vi "tm3samp_06_framerate_wVision.vi"() -> ()   [LabVIEW 2011]
panel:
  out "Display":T1(plugin-control)
  out "Software FPS":dbl
  out "Camera FPS":dbl
  out "Camera Serial":string
  out "Camera Version":string
  out "Camera Model":string
  out "SMD":dbl
  in  "Scan Mode":dbl min=1.0 max=2.0 step=1.0
  in  "Exposure":dbl min=0.0010036691729323308 max=10.000004210526315 step=1e-08
  out "EXP":dbl
  out "SVW":i32
  out "SHW":i32
  out "SVO":i32
  out "SHO":i32
  in  "V Width":i32 min=4 max=1028 step=4
  in  "V Offset":i32 min=0 max=2044 step=4
  in  "H Width":i32 min=4 max=2048 step=4
  in  "H Offset":i32 min=0 max=0 step=4
  in  "Binning":u16(ring)=1 items=["1x1"=1, "2x2"=2, "4x4"=4]
  out "Elapsed Time":u32
  out "Total Frames":i32
  in  "Display":bool=TRUE
  out "error out":errorcluster
  in  "stop":bool
  # "This example displays the frame rate\nof the camera.  Changing the resolution\nof the camera or displaying the images\nwill affect the frame rate."
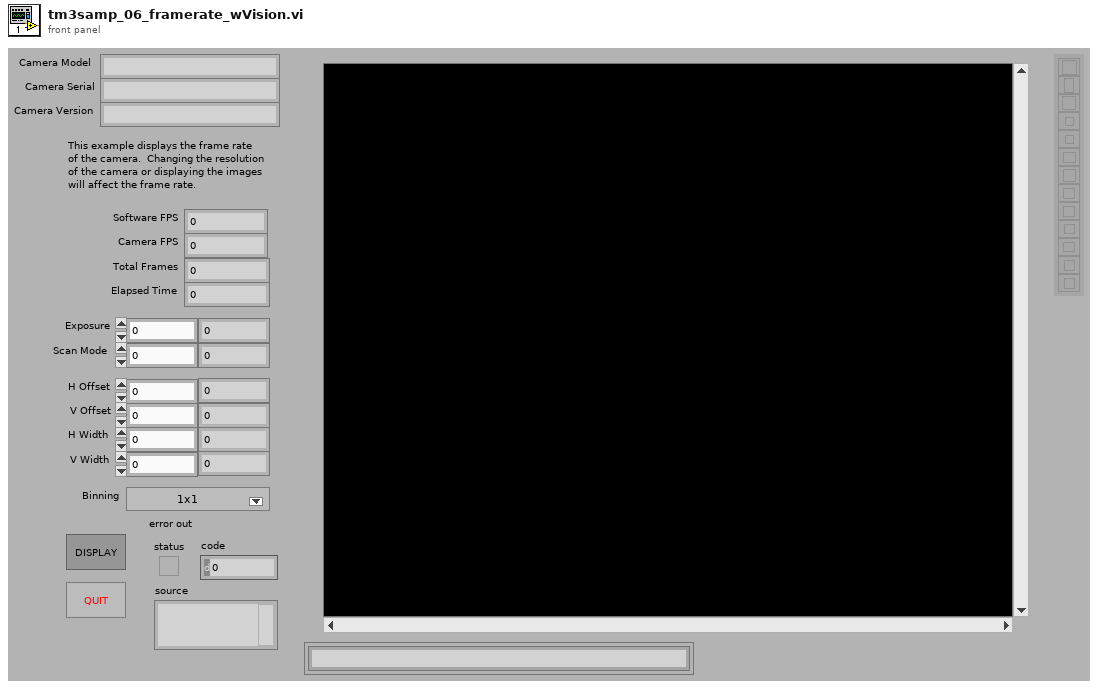
[diagram p1: front panel]
types:
  T1 = typedef "IMAQ Image.ctl" = refnum<image>
  T2 = typedef "Image Type" = u32
  T3 = cluster{"Model":string, "Camera ID":string, "Firmware":string}
  T4 = cluster{"Value":i32, "Minimum":i32, "Maximum":i32, "Increment":i32}
  T5 = cluster{"height":u32, "width":u32, "datatype":u32}
  T6 = cluster{"H Offset":i32, "V Offset":i32, "H Width":i32, "V Width":i32}
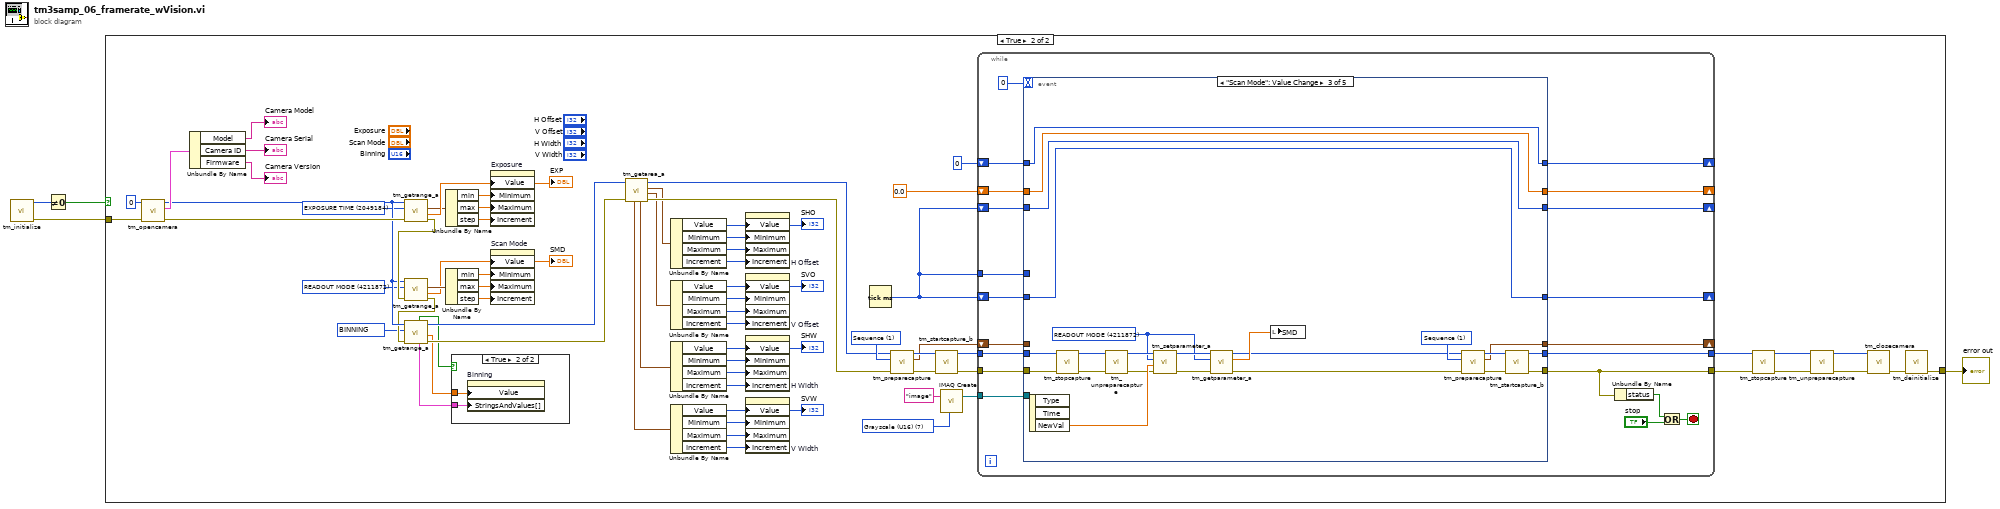
[diagram p0: block diagram]
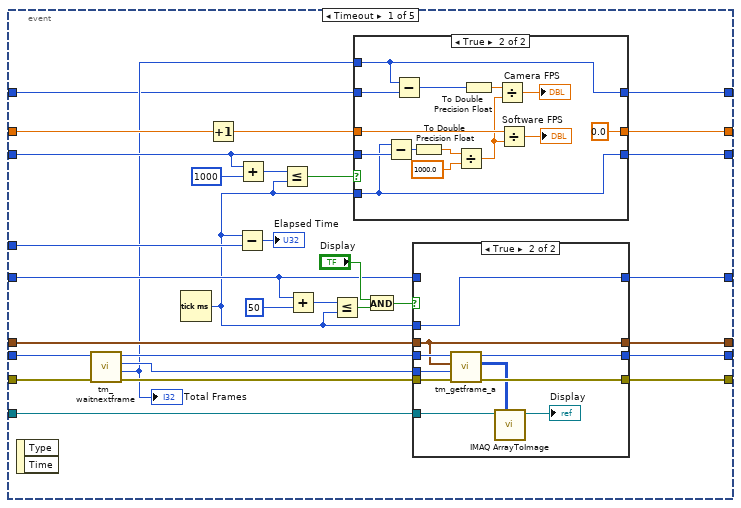
[diagram p4: hidden frame]
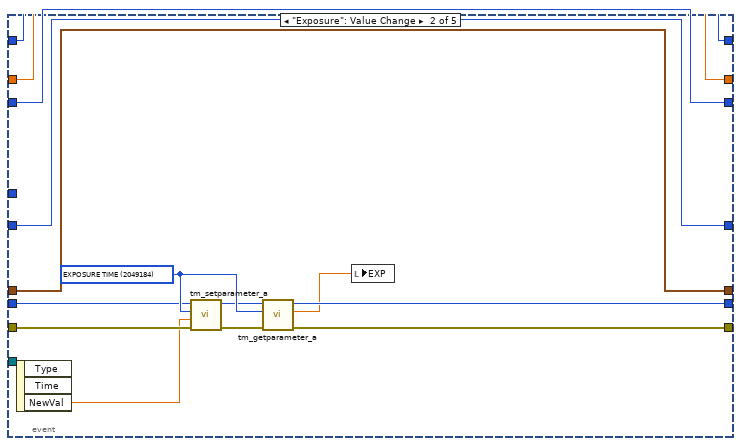
[diagram p7: hidden frame]
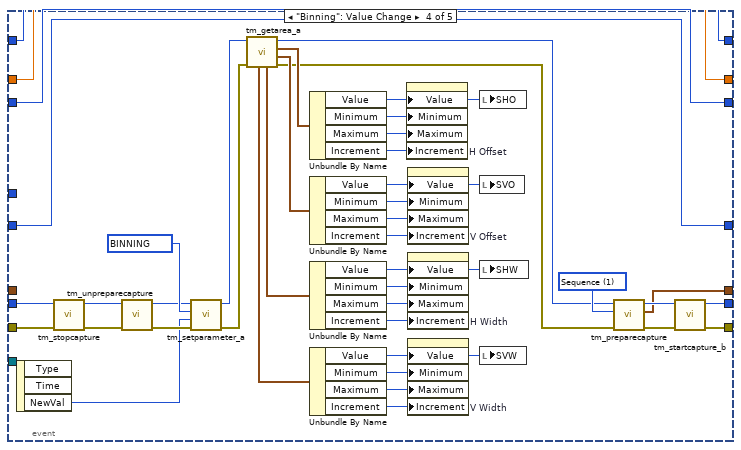
[diagram p8: hidden frame]
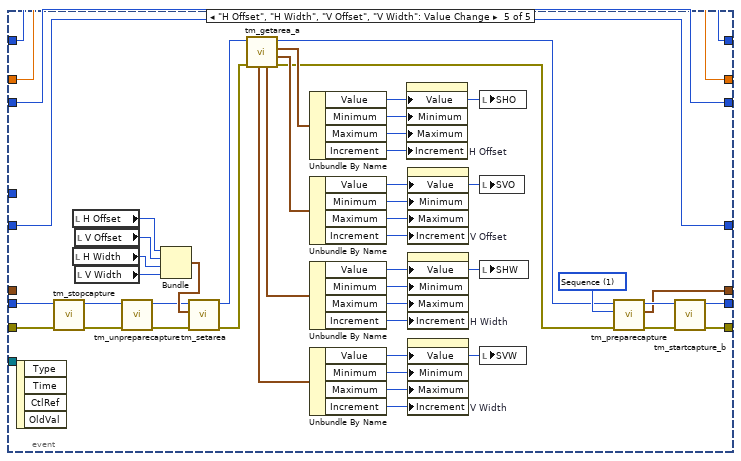
[diagram p9: hidden frame]
diagram:
  n1 = call <userlib>:"tm_initialize.vi"() -> ("error out"=w2:errorcluster, "Number Of Cameras"=w1:u32)  [unwired: 8 in, 2 out]
  n2 = Not Equal To 0?(x=w1) -> (x != 0?=w4:bool)
  n3 = case shown="True" w4 {
    tunnel: [w5 w72] -> w3
    tunnel: w2 -> [w5 w75]
    frame False {
    }
    frame True {
      w7 = T2 7 items=["Grayscale (U8)", "Grayscale (I16)", "Grayscale (SGL)", "Complex (CSG)", "RGB (U32)", "HSL (U32)", "RGB (U64)", "Grayscale (U16)"] ("Image Type")
      w9 = u32 2049184 items=["BINNING"=4215968, "BITS PER CHANNEL"=4342976, "ACTIVE VIEW INDEX"=4343136, "CCD MODE"=4212384, "SENSOR MODE"=4212128, "READOUT MODE"=4211872, "EXPOSURE TIME"=2049184, "CONTRAST GAIN"=3163312, "CONTRAST OFFSET"=3163328, "LIGHT MODE"=2114720, "SENSITIVITY"=2114992, "WHITE BALANCE"=3163568, "PHOTON IMAGING MODE"=2115200, "HIGH DYNAMIC RANGE MODE"=3163360, "TRIGGER SOURCE"=1066144, "TRIGGER ACTIVE"=1066160, "TRIGGER MODE"=1066400, "TRIGGER POLARITY"=1066416, "TRIGGER GLOBAL EXPOSURE"=2049680, "FIRST TRIGGER BEHAVIOR"=2049696, "TRIGGER TIMES"=1066448, "OUTPUT TRIGGER POLARITY"=1852592, "OUTPUT TRIGGER DELAY"=1852624, "OUTPUT TRIGGER PERIOD"=1852640, "TEMPERATURE"=2115232, "TEMPERATURE TARGET"=2115264, "SENSOR COOLER FAN"=2115296, "MECHANICAL SHUTTER"=2115488, "BACK FOCUS POSITION"=8422304, "FRAMEBUNDLE MODE"=4346784, "FRAMEBUNDLE NUMBER"=4346800, "LINEBUNDLE HEIGHT"=4212192, "TRIGGER CONNECTOR"=1066432, "IMAGE PIXEL TYPE"=4343296, "OUTPUT TRIGGER KIND"=1852656, "READOUT DIRECTION"=4211904, "CHANNEL SYNC"=1852352] ("Parameter")
      w10 = u32 4211872 items=["BINNING"=4215968, "BITS PER CHANNEL"=4342976, "ACTIVE VIEW INDEX"=4343136, "CCD MODE"=4212384, "SENSOR MODE"=4212128, "READOUT MODE"=4211872, "EXPOSURE TIME"=2049184, "CONTRAST GAIN"=3163312, "CONTRAST OFFSET"=3163328, "LIGHT MODE"=2114720, "SENSITIVITY"=2114992, "WHITE BALANCE"=3163568, "PHOTON IMAGING MODE"=2115200, "HIGH DYNAMIC RANGE MODE"=3163360, "TRIGGER SOURCE"=1066144, "TRIGGER ACTIVE"=1066160, "TRIGGER MODE"=1066400, "TRIGGER POLARITY"=1066416, "TRIGGER GLOBAL EXPOSURE"=2049680, "FIRST TRIGGER BEHAVIOR"=2049696, "TRIGGER TIMES"=1066448, "OUTPUT TRIGGER POLARITY"=1852592, "OUTPUT TRIGGER DELAY"=1852624, "OUTPUT TRIGGER PERIOD"=1852640, "TEMPERATURE"=2115232, "TEMPERATURE TARGET"=2115264, "SENSOR COOLER FAN"=2115296, "MECHANICAL SHUTTER"=2115488, "BACK FOCUS POSITION"=8422304, "FRAMEBUNDLE MODE"=4346784, "FRAMEBUNDLE NUMBER"=4346800, "LINEBUNDLE HEIGHT"=4212192, "TRIGGER CONNECTOR"=1066432, "IMAGE PIXEL TYPE"=4343296, "OUTPUT TRIGGER KIND"=1852656, "READOUT DIRECTION"=4211904, "CHANNEL SYNC"=1852352] ("Parameter")
      w11 = u32 4215968 items=["BINNING"=4215968, "BITS PER CHANNEL"=4342976, "ACTIVE VIEW INDEX"=4343136, "CCD MODE"=4212384, "SENSOR MODE"=4212128, "READOUT MODE"=4211872, "EXPOSURE TIME"=2049184, "CONTRAST GAIN"=3163312, "CONTRAST OFFSET"=3163328, "LIGHT MODE"=2114720, "SENSITIVITY"=2114992, "WHITE BALANCE"=3163568, "PHOTON IMAGING MODE"=2115200, "HIGH DYNAMIC RANGE MODE"=3163360, "TRIGGER SOURCE"=1066144, "TRIGGER ACTIVE"=1066160, "TRIGGER MODE"=1066400, "TRIGGER POLARITY"=1066416, "TRIGGER GLOBAL EXPOSURE"=2049680, "FIRST TRIGGER BEHAVIOR"=2049696, "TRIGGER TIMES"=1066448, "OUTPUT TRIGGER POLARITY"=1852592, "OUTPUT TRIGGER DELAY"=1852624, "OUTPUT TRIGGER PERIOD"=1852640, "TEMPERATURE"=2115232, "TEMPERATURE TARGET"=2115264, "SENSOR COOLER FAN"=2115296, "MECHANICAL SHUTTER"=2115488, "BACK FOCUS POSITION"=8422304, "FRAMEBUNDLE MODE"=4346784, "FRAMEBUNDLE NUMBER"=4346800, "LINEBUNDLE HEIGHT"=4212192, "TRIGGER CONNECTOR"=1066432, "IMAGE PIXEL TYPE"=4343296, "OUTPUT TRIGGER KIND"=1852656, "READOUT DIRECTION"=4211904, "CHANNEL SYNC"=1852352] ("Parameter")
      w70 = 1 items=["Snap", "Sequence"] ("Capture mode")
      n4 = call <userlib>:"tm_opencamera.vi"("error in (no error)"=w75, "Camera Index"=u32 0) -> ("error out"=w24:errorcluster, "Camera Details"=w28:T3, "Handle out"=w18:u32)  [unwired: 7 in]
      n5 = Unbundle By Name(w28) -> ("Model"=→"Camera Model":string, "Camera ID"=→"Camera Serial":string, "Firmware"=→"Camera Version":string)
      n6 = call <userlib>:"tm_getrange_a.vi"("error in (no error)"=w24, "Parameter"=w9, "Handle in"=w18) -> ("error out"=w21:errorcluster, "default"=w23:dbl, "Range"=w22:cluster{"min":dbl, "max":dbl, "step":dbl})  [unwired: 2 in, 4 out]
      "EXP" <- w23
      n7 = call <userlib>:"tm_getrange_a.vi"("error in (no error)"=w21, "Parameter"=w10, "Handle in"=w18) -> ("error out"=w17:errorcluster, "default"=w19:dbl, "Range"=w20:cluster{"min":dbl, "max":dbl, "step":dbl})  [unwired: 2 in, 4 out]
      "SMD" <- w19
      n8 = call <userlib>:"tm_getrange_a.vi"("error in (no error)"=w17, "Parameter"=w11, "Handle in"=w18) -> ("error out"=w16:errorcluster, "default"=w13:dbl, "Handle out"=w15:u32, "Value Names"=w12:cluster{"Name":string, "Value":dbl}[], "Writable"=w14:bool)  [unwired: 2 in, 2 out]
      n9 = Unbundle By Name(w22) -> ("min"=w63:dbl, "max"=w62:dbl, "step"=w61:dbl)
      n10 = Unbundle By Name(w20) -> ("min"=w60:dbl, "max"=w59:dbl, "step"=w58:dbl)
      n11 = case shown="True" w14 {
        tunnel: w12 -> [_ w77]
        tunnel: w13 -> [_ w76]
        frame False {
        }
        frame True {
          n12 = property on="Binning" class="Ring (strict)"("Value"=w76, "StringsAndValues[]"=w77) -> ()  [unwired: 2 in, 2 out]
        }
      }
      n13 = property on="Exposure" class="DigNum (strict)"("Value"=w23, "Minimum"=w63, "Maximum"=w62, "Increment"=w61) -> ()  [unwired: 2 in, 2 out]
      n14 = property on="Scan Mode" class="DigNum (strict)"("Value"=w19, "Minimum"=w60, "Maximum"=w59, "Increment"=w58) -> ()  [unwired: 2 in, 2 out]
      n15 = call <userlib>:"tm_getarea_a.vi"("error in (no error)"=w16, "Handle in"=w15) -> ("error out"=w56:errorcluster, "V Offset"=w55:T4, "H Offset"=w34:T4, "Handle out"=w57:u32, "H Width"=w54:T4, "V Width"=w53:T4)  [unwired: 4 in]
      n16 = Unbundle By Name(w34) -> ("Value"=w33:i32, "Minimum"=w32:i32, "Maximum"=w31:i32, "Increment"=w30:i32)
      "SHO" <- w33
      n17 = Unbundle By Name(w55) -> ("Value"=w43:i32, "Minimum"=w52:i32, "Maximum"=w51:i32, "Increment"=w50:i32)
      "SVO" <- w43
      n18 = Unbundle By Name(w54) -> ("Value"=w42:i32, "Minimum"=w49:i32, "Maximum"=w48:i32, "Increment"=w47:i32)
      "SHW" <- w42
      n19 = Unbundle By Name(w53) -> ("Value"=w41:i32, "Minimum"=w46:i32, "Maximum"=w45:i32, "Increment"=w44:i32)
      "SVW" <- w41
      n20 = property on="H Offset" class="DigNum (strict)"("Value"=w33, "Minimum"=w32, "Maximum"=w31, "Increment"=w30) -> ()  [unwired: 2 in, 2 out]
      n21 = property on="V Offset" class="DigNum (strict)"("Value"=w43, "Minimum"=w52, "Maximum"=w51, "Increment"=w50) -> ()  [unwired: 2 in, 2 out]
      n22 = property on="H Width" class="DigNum (strict)"("Value"=w42, "Minimum"=w49, "Maximum"=w48, "Increment"=w47) -> ()  [unwired: 2 in, 2 out]
      n23 = property on="V Width" class="DigNum (strict)"("Value"=w41, "Minimum"=w46, "Maximum"=w45, "Increment"=w44) -> ()  [unwired: 2 in, 2 out]
      n24 = Tick Count (ms)() -> (millisecond timer value=w64:u32)
      n25 = call <userlib>:"tm_preparecapture.vi"("error in (no error)"=w56, "Capture mode"=w70, "Handle in"=w57) -> ("error out"=w68:errorcluster, "Buffer Info"=w65:T5, "Handle out"=w69:u32)  [unwired: 5 in, 1 out]
      n26 = call <userlib>:"tm_startcapture_b.vi"("error in (no error)"=w68, "Handle in"=w69) -> ("error out"=w67:errorcluster, "Handle out"=w66:u32)  [unwired: 8 in]
      n27 = call "IMAQ Create"("Image Name"="image", "Image Type"=w7) -> ("New Image"=w6:T1)  [unwired: 3 in, 1 out]
      n28 = while {
        tunnel: w67 -> [w86]
        tunnel: [w84] -> w40
        tunnel: [w83] -> w39
        shift-right: [w93] -> _
        shift-left: w64 -> [w91]
        shift-right: [w94] -> _
        shift-left: 0.0 -> [w92]
        shift-right: [w85] -> _
        shift-left: w64 -> [w89]
        tunnel: w66 -> [w87]
        tunnel: w64 -> [w90]
        shift-right: [w82] -> _
        shift-left: w65 -> [w88]
        shift-right: [w79] -> _
        shift-left: 0 -> [w80]
        tunnel: w6 -> [w78]
        stop <- w95 stop-if-true
        n29 = event shown="[2] \"Scan Mode\": Value Change" {
          selector: _ -> [_ _ _ _ _]
          dyn-events: _ -> [_ _ _ _ _]
          timeout: 0 -> [_ _ _ _ _]
          tunnel: [w103 w171 w194 w230 w275] -> w94
          tunnel: [w102 w172 w195 w231 w276] -> w93
          tunnel: w92 -> [w114 w171 w194 w230 w275]
          tunnel: w91 -> [w105 w172 w195 w231 w276]
          tunnel: w90 -> [w110 _ _ _ _]
          tunnel: w89 -> [w115 w173 w196 w238 w283]
          tunnel: w88 -> [w109 w170 _ _ _]
          tunnel: w87 -> [w117 w165 w191 w207 w245]
          tunnel: w86 -> [w116 w167 w190 w206 w244]
          tunnel: [w113 w173 w196 w238 w283] -> w85
          tunnel: [w112 w162 w185 w233 w278] -> w84
          tunnel: [w111 w160 w186 w234 w279] -> w83
          tunnel: [w108 w170 w184 w232 w277] -> w82
          tunnel: w80 -> [w100 w169 w183 w203 w239]
          tunnel: [w99 w169 w183 w203 w239] -> w79
          tunnel: w78 -> [w98 _ _ _ _]
          event Timeout {
            n30 = event-data() -> ()  [unwired: 1 in, 2 out]
            n31 = call <userlib>:"tm_waitnextframe.vi"("error in (no error)"=w116, "Handle in"=w117) -> ("error out"=w121:errorcluster, "Frame Count"=w101:i32, "Frame Index"=w120:i32, "Handle out"=w122:u32)  [unwired: 6 in]
            "Total Frames" <- w101
            n32 = Tick Count (ms)() -> (millisecond timer value=w107:u32)
            n33 = Increment(x=w114) -> (x+1=w104:dbl)
            n34 = Subtract(x=w107, y=w110) -> (x-y=→"Elapsed Time":u32)
            n35 = Add(x=w105, y=u32 1000) -> (x+y=w128:u32)
            n36 = Less Or Equal?(x=w128, y=w107) -> (x <= y?=w106:bool)
            n37 = Add(x=w115, y=u32 50) -> (x+y=w126:u32)
            n38 = Less Or Equal?(x=w126, y=w107) -> (x <= y?=w124:bool)
            n39 = case shown="True" w106 {
              tunnel: w105 -> [w131 w140]
              tunnel: [w131 w137] -> w102
              tunnel: w104 -> [w130 w143]
              tunnel: w107 -> [_ w137]
              tunnel: [w130 0.0] -> w103
              tunnel: w101 -> [_ w132]
              tunnel: w100 -> [w129 w135]
              tunnel: [w129 w132] -> w99
              frame False {
              }
              frame True {
                n40 = Subtract(x=w137, y=w140) -> (x-y=w139:u32)
                n41 = Subtract(x=w132, y=w135) -> (x-y=w133:i32)
                n42 = To Double Precision Float(number=w139) -> (double precision float=w145:dbl)
                n43 = Divide(x=w145, y=1000.0) -> (x/y=w136:dbl)
                n44 = To Double Precision Float(number=w133) -> (double precision float=w134:dbl)
                n45 = Divide(x=w134, y=w136) -> (x/y=→"Camera FPS":dbl)
                n46 = Divide(x=w143, y=w136) -> (x/y=→"Software FPS":dbl)
              }
            }
            n47 = And(x="Display", y=w124) -> (x .and. y?=w119:bool)
            n48 = case shown="True" w119 {
              tunnel: w115 -> [w149 _]
              tunnel: w107 -> [_ w159]
              tunnel: [w149 w159] -> w113
              tunnel: w122 -> [w148 w158]
              tunnel: w109 -> [w146 w153]
              tunnel: w121 -> [w147 w157]
              tunnel: [w148 w156] -> w112
              tunnel: [w147 w155] -> w111
              tunnel: w120 -> [_ w154]
              tunnel: [w146 w153] -> w108
              tunnel: w98 -> [_ w151]
              frame False {
              }
              frame True {
                n49 = call <userlib>:"tm_getframe_a.vi"("error in (no error)"=w157, "Frame Index"=w154, "Buffer Info"=w153, "Handle in"=w158) -> ("error out"=w155:errorcluster, "Data 16"=w152:u16[][], "Handle out"=w156:u32)  [unwired: 3 in, 2 out]
                n50 = call "IMAQ ArrayToImage"("Image Pixels (U16)"=w152, "Image"=w151) -> ("Image Out"=→"Display":T1)  [unwired: 8 in, 1 out]
              }
            }
          }
          event "Exposure": Value Change {
            w168 = u32 2049184 items=["SENSOR MODE"=4212128, "CCD MODE"=4212384, "READOUT MODE"=4211872, "ACTIVE VIEW INDEX"=4343136, "BITS PER CHANNEL"=4342976, "IMAGE PIXEL TYPE"=4343296, "BINNING"=4215968, "EXPOSURE TIME"=2049184, "CONTRAST GAIN"=3163312, "CONTRAST OFFSET"=3163328, "LIGHT MODE"=2114720, "SENSITIVITY"=2114992, "PHOTON IMAGING MODE"=2115200, "HIGH DYNAMIC RANGE MODE"=3163360, "WHITE BALANCE"=3163568, "TEMPERATURE"=2115232, "TEMPERATURE TARGET"=2115264, "SENSOR COOLER FAN"=2115296, "LINEBUNDLE HEIGHT"=4212192, "MECHANICAL SHUTTER"=2115488, "BACK FOCUS POSITION"=8422304, "TRIGGER CONNECTOR"=1066432, "TRIGGER SOURCE"=1066144, "OUTPUT TRIGGER SOURCE"=1852576, "TRIGGER GLOBAL EXPOSURE"=2049680, "FIRST TRIGGER BEHAVIOR"=2049696, "CHANNEL SYNC"=1852352, "READOUT DIRECTION"=4211904, "PRE HSYNC COUNT"=1852704] ("Parameter")
            n51 = event-data() -> ("NewVal"=w166:dbl)  [unwired: 1 in, 2 out]
            n52 = call <userlib>:"tm_setparameter_a.vi"("error in (no error)"=w167, "Value in"=w166, "Parameter"=w168, "Handle in"=w165) -> ("error out"=w164:errorcluster, "Handle out"=w163:u32)  [unwired: 6 in]
            n53 = call <userlib>:"tm_getparameter_a.vi"("error in (no error)"=w164, "Parameter"=w168, "Handle in"=w163) -> ("error out"=w160:errorcluster, "Value out"=w161:dbl, "Handle out"=w162:u32)  [unwired: 6 in]
            n54 = local write "EXP"(w161) -> ()
          }
          event "Scan Mode": Value Change {
            w174 = u32 4211872 items=["SENSOR MODE"=4212128, "CCD MODE"=4212384, "READOUT MODE"=4211872, "ACTIVE VIEW INDEX"=4343136, "BITS PER CHANNEL"=4342976, "IMAGE PIXEL TYPE"=4343296, "BINNING"=4215968, "EXPOSURE TIME"=2049184, "CONTRAST GAIN"=3163312, "CONTRAST OFFSET"=3163328, "LIGHT MODE"=2114720, "SENSITIVITY"=2114992, "PHOTON IMAGING MODE"=2115200, "HIGH DYNAMIC RANGE MODE"=3163360, "WHITE BALANCE"=3163568, "TEMPERATURE"=2115232, "TEMPERATURE TARGET"=2115264, "SENSOR COOLER FAN"=2115296, "LINEBUNDLE HEIGHT"=4212192, "MECHANICAL SHUTTER"=2115488, "BACK FOCUS POSITION"=8422304, "TRIGGER CONNECTOR"=1066432, "TRIGGER SOURCE"=1066144, "OUTPUT TRIGGER SOURCE"=1852576, "TRIGGER GLOBAL EXPOSURE"=2049680, "FIRST TRIGGER BEHAVIOR"=2049696, "CHANNEL SYNC"=1852352, "READOUT DIRECTION"=4211904, "PRE HSYNC COUNT"=1852704] ("Parameter")
            w189 = 1 items=["Snap", "Sequence"] ("Capture mode")
            n55 = event-data() -> ("NewVal"=w179:dbl)  [unwired: 1 in, 2 out]
            n56 = call <userlib>:"tm_stopcapture.vi"("error in (no error)"=w190, "Handle in"=w191) -> ("error out"=w192:errorcluster, "Handle out"=w193:u32)  [unwired: 8 in]
            n57 = call <userlib>:"tm_unpreparecapture.vi"("error in (no error)"=w192, "Handle in"=w193) -> ("error out"=w177:errorcluster, "Handle out"=w178:u32)  [unwired: 8 in]
            n58 = call <userlib>:"tm_setparameter_a.vi"("error in (no error)"=w177, "Value in"=w179, "Parameter"=w174, "Handle in"=w178) -> ("error out"=w176:errorcluster, "Handle out"=w175:u32)  [unwired: 6 in]
            n59 = call <userlib>:"tm_getparameter_a.vi"("error in (no error)"=w176, "Parameter"=w174, "Handle in"=w175) -> ("error out"=w182:errorcluster, "Value out"=w181:dbl, "Handle out"=w180:u32)  [unwired: 6 in]
            n60 = local write "SMD"(w181) -> ()
            n61 = call <userlib>:"tm_preparecapture.vi"("error in (no error)"=w182, "Capture mode"=w189, "Handle in"=w180) -> ("error out"=w187:errorcluster, "Buffer Info"=w184:T5, "Handle out"=w188:u32)  [unwired: 5 in, 1 out]
            n62 = call <userlib>:"tm_startcapture_b.vi"("error in (no error)"=w187, "Handle in"=w188) -> ("error out"=w186:errorcluster, "Handle out"=w185:u32)  [unwired: 8 in]
          }
          event "Binning": Value Change {
            w198 = u32 4215968 items=["BINNING"=4215968, "BITS PER CHANNEL"=2, "ACTIVE VIEW INDEX"=3, "CCD MODE"=4, "SENSOR MODE"=5, "READOUT MODE"=6, "EXPOSURE TIME"=7, "CONTRAST GAIN"=8, "CONTRAST OFFSET"=9, "LIGHT MODE"=10, "SENSITIVITY"=11, "WHITE BALANCE"=12, "PHOTON IMAGING MODE"=13, "HIGH DYNAMIC RANGE MODE"=14, "TRIGGER SOURCE"=15, "TRIGGER ACTIVE"=16, "TRIGGER MODE"=17, "TRIGGER POLARITY"=18, "TRIGGER GLOBAL EXPOSURE"=19, "FIRST TRIGGER BEHAVIOR"=20, "TRIGGER TIMES"=21, "OUTPUT TRIGGER POLARITY"=22, "OUTPUT TRIGGER DELAY"=23, "OUTPUT TRIGGER PERIOD"=24, "TEMPERATURE"=25, "TEMPERATURE TARGET"=26, "SENSOR COOLER FAN"=27, "MECHANICAL SHUTTER"=28, "BACK FOCUS POSITION"=29, "FRAMEBUNDLE MODE"=30, "FRAMEBUNDLE NUMBER"=31, "LINEBUNDLE HEIGHT"=32, "TRIGGER CONNECTOR"=33, "IMAGE PIXEL TYPE"=34, "OUTPUT TRIGGER KIND"=35, "READOUT DIRECTION"=36, "CHANNEL SYNC"=37] ("Parameter")
            w237 = 1 items=["Snap", "Sequence"] ("Capture mode")
            n63 = event-data() -> ("NewVal"=w199:u16)  [unwired: 1 in, 2 out]
            n64 = call <userlib>:"tm_stopcapture.vi"("error in (no error)"=w206, "Handle in"=w207) -> ("error out"=w204:errorcluster, "Handle out"=w205:u32)  [unwired: 8 in]
            n65 = call <userlib>:"tm_unpreparecapture.vi"("error in (no error)"=w204, "Handle in"=w205) -> ("error out"=w200:errorcluster, "Handle out"=w197:u32)  [unwired: 8 in]
            n66 = call <userlib>:"tm_setparameter_a.vi"("error in (no error)"=w200, "Value in"=w199, "Parameter"=w198, "Handle in"=w197) -> ("error out"=w201:errorcluster, "Handle out"=w202:u32)  [unwired: 6 in]
            n67 = call <userlib>:"tm_getarea_a.vi"("error in (no error)"=w201, "Handle in"=w202) -> ("error out"=w225:errorcluster, "V Offset"=w227:T4, "H Offset"=w226:T4, "Handle out"=w224:u32, "H Width"=w228:T4, "V Width"=w229:T4)  [unwired: 4 in]
            n68 = Unbundle By Name(w226) -> ("Value"=w220:i32, "Minimum"=w223:i32, "Maximum"=w222:i32, "Increment"=w221:i32)
            n69 = Unbundle By Name(w227) -> ("Value"=w210:i32, "Minimum"=w219:i32, "Maximum"=w218:i32, "Increment"=w217:i32)
            n70 = Unbundle By Name(w228) -> ("Value"=w209:i32, "Minimum"=w216:i32, "Maximum"=w215:i32, "Increment"=w214:i32)
            n71 = Unbundle By Name(w229) -> ("Value"=w208:i32, "Minimum"=w213:i32, "Maximum"=w212:i32, "Increment"=w211:i32)
            n72 = property on="H Offset" class="DigNum (strict)"("Value"=w220, "Minimum"=w223, "Maximum"=w222, "Increment"=w221) -> ()  [unwired: 2 in, 2 out]
            n73 = property on="V Offset" class="DigNum (strict)"("Value"=w210, "Minimum"=w219, "Maximum"=w218, "Increment"=w217) -> ()  [unwired: 2 in, 2 out]
            n74 = property on="H Width" class="DigNum (strict)"("Value"=w209, "Minimum"=w216, "Maximum"=w215, "Increment"=w214) -> ()  [unwired: 2 in, 2 out]
            n75 = property on="V Width" class="DigNum (strict)"("Value"=w208, "Minimum"=w213, "Maximum"=w212, "Increment"=w211) -> ()  [unwired: 2 in, 2 out]
            n76 = local write "SHO"(w220) -> ()
            n77 = local write "SVO"(w210) -> ()
            n78 = local write "SHW"(w209) -> ()
            n79 = local write "SVW"(w208) -> ()
            n80 = call <userlib>:"tm_preparecapture.vi"("error in (no error)"=w225, "Capture mode"=w237, "Handle in"=w224) -> ("error out"=w235:errorcluster, "Buffer Info"=w232:T5, "Handle out"=w236:u32)  [unwired: 5 in, 1 out]
            n81 = call <userlib>:"tm_startcapture_b.vi"("error in (no error)"=w235, "Handle in"=w236) -> ("error out"=w234:errorcluster, "Handle out"=w233:u32)  [unwired: 8 in]
          }
          event "H Offset", "H Width", "V Offset", "V Width": Value Change {
            w282 = 1 items=["Snap", "Sequence"] ("Capture mode")
            n82 = event-data() -> ()  [unwired: 1 in, 4 out]
            n83 = call <userlib>:"tm_stopcapture.vi"("error in (no error)"=w244, "Handle in"=w245) -> ("error out"=w242:errorcluster, "Handle out"=w243:u32)  [unwired: 8 in]
            n84 = local read "H Offset"() -> (w248:i32)
            n85 = local read "H Width"() -> (w249:i32)
            n86 = local read "V Offset"() -> (w250:i32)
            n87 = local read "V Width"() -> (w247:i32)
            n88 = call <userlib>:"tm_unpreparecapture.vi"("error in (no error)"=w242, "Handle in"=w243) -> ("error out"=w240:errorcluster, "Handle out"=w241:u32)  [unwired: 8 in]
            n89 = Bundle("H Offset"=w248, "V Offset"=w250, "H Width"=w249, "V Width"=w247) -> (w246:T6)  [unwired: 1 in]
            n90 = call <userlib>:"tm_setarea.vi"("error in (no error)"=w240, "Sub Region"=w246, "Handle in"=w241) -> ("error out"=w251:errorcluster, "Handle out"=w252:u32)  [unwired: 7 in]
            n91 = call <userlib>:"tm_getarea_a.vi"("error in (no error)"=w251, "Handle in"=w252) -> ("error out"=w270:errorcluster, "V Offset"=w272:T4, "H Offset"=w271:T4, "Handle out"=w269:u32, "H Width"=w273:T4, "V Width"=w274:T4)  [unwired: 4 in]
            n92 = Unbundle By Name(w271) -> ("Value"=w265:i32, "Minimum"=w268:i32, "Maximum"=w267:i32, "Increment"=w266:i32)
            n93 = Unbundle By Name(w272) -> ("Value"=w255:i32, "Minimum"=w264:i32, "Maximum"=w263:i32, "Increment"=w262:i32)
            n94 = Unbundle By Name(w273) -> ("Value"=w254:i32, "Minimum"=w261:i32, "Maximum"=w260:i32, "Increment"=w259:i32)
            n95 = Unbundle By Name(w274) -> ("Value"=w253:i32, "Minimum"=w258:i32, "Maximum"=w257:i32, "Increment"=w256:i32)
            n96 = property on="H Offset" class="DigNum (strict)"("Value"=w265, "Minimum"=w268, "Maximum"=w267, "Increment"=w266) -> ()  [unwired: 2 in, 2 out]
            n97 = property on="V Offset" class="DigNum (strict)"("Value"=w255, "Minimum"=w264, "Maximum"=w263, "Increment"=w262) -> ()  [unwired: 2 in, 2 out]
            n98 = property on="H Width" class="DigNum (strict)"("Value"=w254, "Minimum"=w261, "Maximum"=w260, "Increment"=w259) -> ()  [unwired: 2 in, 2 out]
            n99 = property on="V Width" class="DigNum (strict)"("Value"=w253, "Minimum"=w258, "Maximum"=w257, "Increment"=w256) -> ()  [unwired: 2 in, 2 out]
            n100 = local write "SHO"(w265) -> ()
            n101 = local write "SVO"(w255) -> ()
            n102 = local write "SHW"(w254) -> ()
            n103 = local write "SVW"(w253) -> ()
            n104 = call <userlib>:"tm_preparecapture.vi"("error in (no error)"=w270, "Capture mode"=w282, "Handle in"=w269) -> ("error out"=w280:errorcluster, "Buffer Info"=w277:T5, "Handle out"=w281:u32)  [unwired: 5 in, 1 out]
            n105 = call <userlib>:"tm_startcapture_b.vi"("error in (no error)"=w280, "Handle in"=w281) -> ("error out"=w279:errorcluster, "Handle out"=w278:u32)  [unwired: 8 in]
          }
        }
        n106 = Unbundle By Name(w83) -> ("status"=w96:bool)
        n107 = Or(x=w96, y="stop") -> (x .or. y?=w95:bool)
      }
      n108 = call <userlib>:"tm_stopcapture.vi"("error in (no error)"=w39, "Handle in"=w40) -> ("error out"=w36:errorcluster, "Handle out"=w37:u32)  [unwired: 8 in]
      n109 = call <userlib>:"tm_unpreparecapture.vi"("error in (no error)"=w36, "Handle in"=w37) -> ("error out"=w35:errorcluster, "Handle out"=w38:u32)  [unwired: 8 in]
      n110 = call <userlib>:"tm_closecamera.vi"("error in (no error)"=w35, "Handle in"=w38) -> ("error out"=w73:errorcluster)  [unwired: 9 in]
      n111 = call <userlib>:"tm_deinitialize.vi"("error in (no error)"=w73) -> ("error out"=w72:errorcluster)  [unwired: 10 in]
    }
  }
  "error out" <- w3
